vi "Holamundo.vi"() -> ()   [LabVIEW 2020]
panel:
  out "Tank 2":dbl(slide) scale=0.0..200.0
  in  "Thermometer":dbl(slide) scale=0.0..100.0
  in  "Vertical Progress Bar":dbl(slide) scale=0.0..100.0
  in  "STOP":bool
  # "control\nindicador"
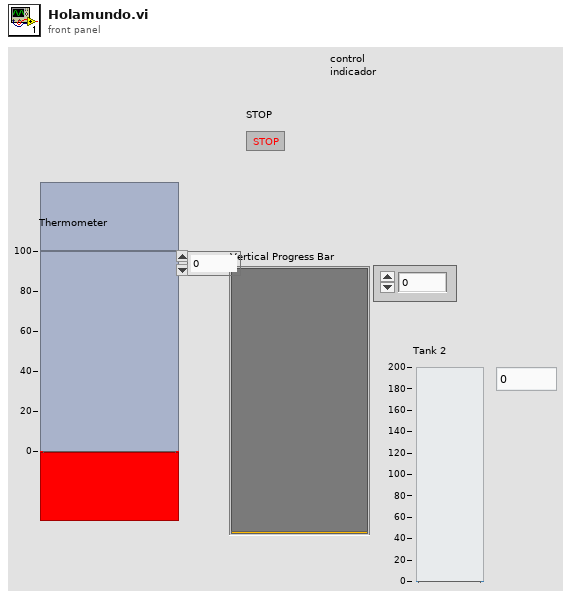
[diagram p1: front panel]
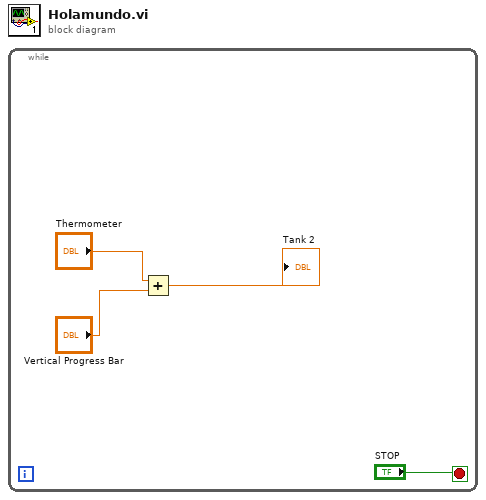
[diagram p0: block diagram]
diagram:
  n1 = while {
    stop <- "STOP" stop-if-true
    n2 = Add(x="Thermometer", y="Vertical Progress Bar") -> (x+y=→"Tank 2":dbl)
  }
